vi "Destroy to SFTP.vi"(8 "Error In":errorcluster, 10 "SFTP Attributes":refnum<class "SFTP Attributes.lvclass">, 11 "SFTP In":refnum<class "SFTP.lvclass">) -> (0 "Error Out":errorcluster, 3 "SFTP Out":refnum<class "SFTP.lvclass">)   [LabVIEW 2018, in "Toolkit.lvlib" / "SFTP Attributes.lvclass"]
uses:
  SFTP Attributes.lvclass
  SFTP/SFTP.lvclass
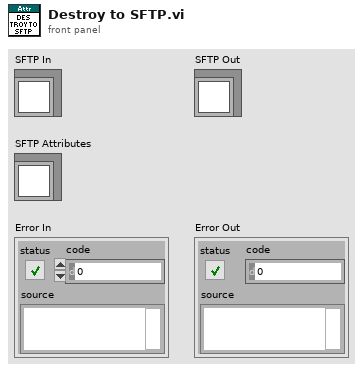
[diagram p1: front panel]
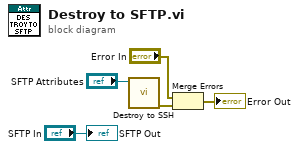
[diagram p0: block diagram]
diagram:
  n1 = call "Destroy to SSH.vi"("SFTP Attributes"="SFTP Attributes") -> ("Error Out"=w2:errorcluster)  [unwired: 9 in, 1 out]
  n2 = Merge Errors("Error In", w2) -> (→"Error Out":errorcluster)
  "SFTP Out" <- "SFTP In"
